vi "Check.vi"() -> ()   [LabVIEW 2023]
uses:
  <vilib>/DAQmx/read.llb/DAQmx Read (Digital Bool 1Line 1Point).vi
  <vilib>/DAQmx/write.llb/DAQmx Write (Digital Bool 1Line 1Point).vi
  <vilib>/DAQmx/read.llb/DAQmx Read (Digital 1D Bool NChan 1Samp 1Line).vi
  <vilib>/Utility/error.llb/Trim Whitespace One-Sided.vi
  <vilib>/DAQmx/create/channels.llb/DAQmx Create Channel (DO-Digital Output).vi
  <vilib>/DAQmx/create/channels.llb/DAQmx Create Channel (DI-Digital Input).vi
  <vilib>/Instr/_visa.llb/VISA Configure Serial Port (Instr).vi
  <vilib>/DAQmx/miscellaneous.llb/DAQmx Fill In Error Info.vi
panel:
  in  "VISA resource name":refnum<visa-resource-name>
  in  "Cry":tag
  in  "Motor":tag
  in  "Available":tag
  in  "Fan":tag
  in  "Wet":tag
  in  "Buzzer":tag
  in  "stop":bool
  in  "Cradle":bool
  out "read buffer":string
  out "Humidity":dbl(slide) scale=0.0..100.0
  out "Temperature":dbl(slide) scale=0.0..100.0
  out "Cry":bool
  out "Available":bool
  out "Wet":bool
  # "Input Output Panel"
  # "Indication Panel"
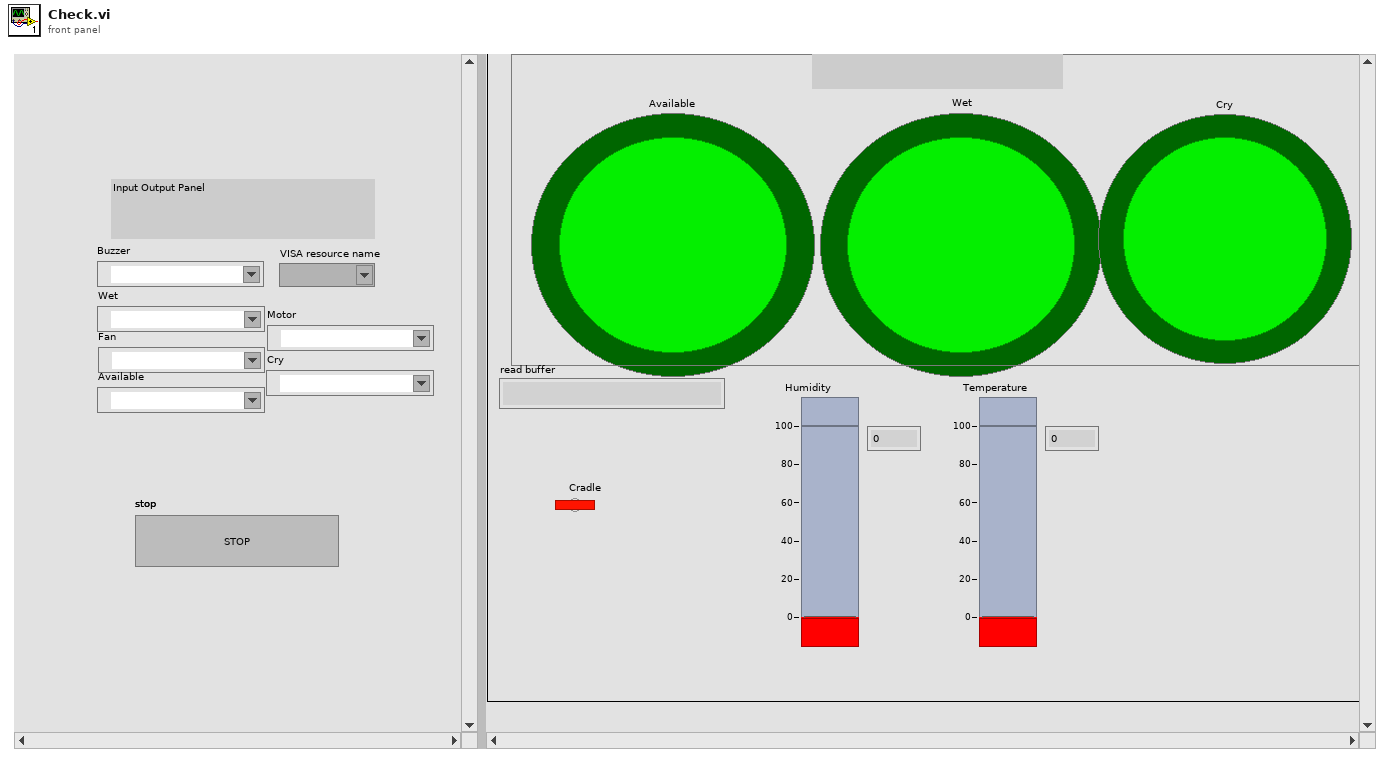
[diagram p1: front panel]
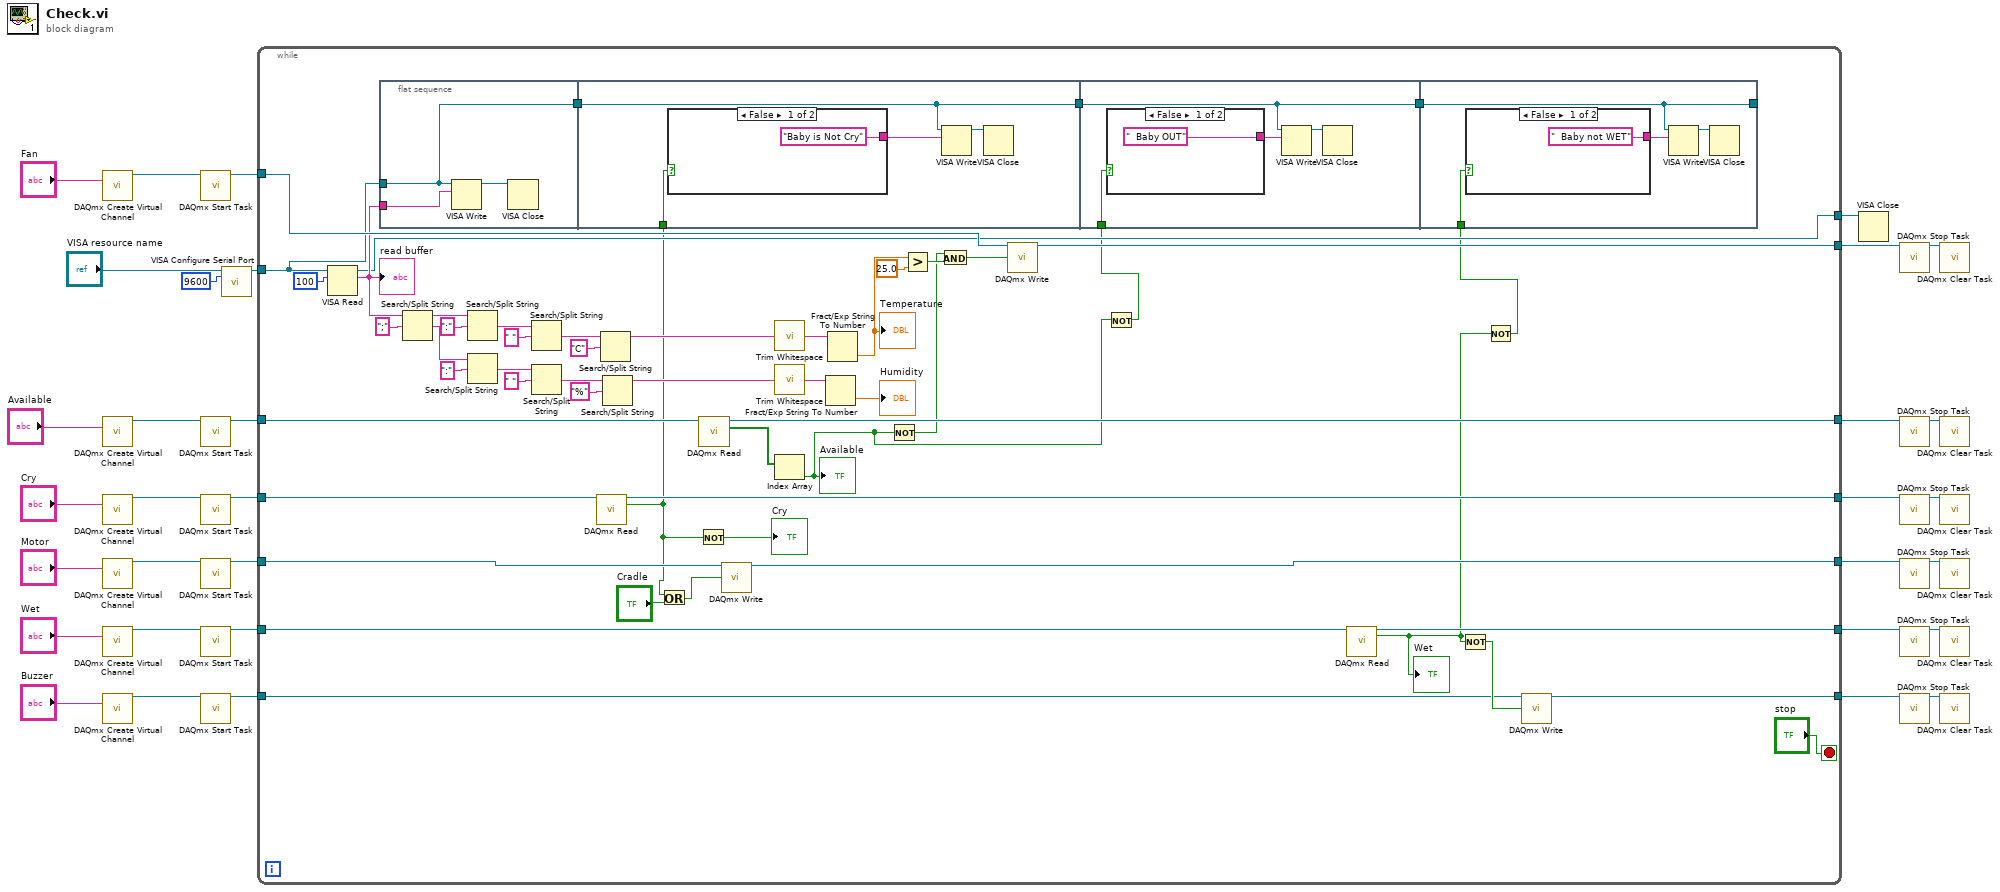
[diagram p0: block diagram]
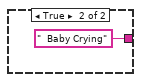
[diagram p2: hidden frame]
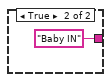
[diagram p3: hidden frame]
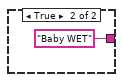
[diagram p4: hidden frame]
diagram:
  n1 = call-poly <vilib>:"DAQmx Create Virtual Channel.vi"("lines"="Fan") -> ("task out"=w21:refnum<k21>)  [unwired: 13 in, 1 out]
  n2 = call-poly <vilib>:"DAQmx Create Virtual Channel.vi"("lines"="Available") -> ("task out"=w18:refnum<k21>)  [unwired: 13 in, 1 out]
  n3 = call-poly <vilib>:"DAQmx Create Virtual Channel.vi"("lines"="Cry") -> ("task out"=w15:refnum<k21>)  [unwired: 13 in, 1 out]
  n4 = call-poly <vilib>:"DAQmx Create Virtual Channel.vi"("lines"="Motor") -> ("task out"=w12:refnum<k21>)  [unwired: 13 in, 1 out]
  n5 = call-poly <vilib>:"DAQmx Create Virtual Channel.vi"("lines"="Wet") -> ("task out"=w30:refnum<k21>)  [unwired: 13 in, 1 out]
  n6 = call-poly <vilib>:"DAQmx Create Virtual Channel.vi"("lines"="Buzzer") -> ("task out"=w34:refnum<k21>)  [unwired: 13 in, 1 out]
  n7 = call <vilib>:"DAQmx Start Task.vi"("task/channels in"=w21) -> ("task out"=w20:refnum<k21>)  [unwired: 13 in, 1 out]
  n8 = call <vilib>:"DAQmx Start Task.vi"("task/channels in"=w18) -> ("task out"=w17:refnum<k21>)  [unwired: 13 in, 1 out]
  n9 = call <vilib>:"DAQmx Start Task.vi"("task/channels in"=w15) -> ("task out"=w14:refnum<k21>)  [unwired: 13 in, 1 out]
  n10 = call <vilib>:"DAQmx Start Task.vi"("task/channels in"=w12) -> ("task out"=w11:refnum<k21>)  [unwired: 13 in, 1 out]
  n11 = call <vilib>:"DAQmx Start Task.vi"("task/channels in"=w30) -> ("task out"=w29:refnum<k21>)  [unwired: 13 in, 1 out]
  n12 = call <vilib>:"DAQmx Start Task.vi"("task/channels in"=w34) -> ("task out"=w2:refnum<k21>)  [unwired: 13 in, 1 out]
  n13 = call-poly "VISA Configure Serial Port"("VISA resource name"="VISA resource name", "baud rate (9600)"=u32 9600) -> ("VISA resource name out"=w4:refnum<visa-resource-name>)  [unwired: 12 in, 1 out]
  n14 = while {
    tunnel: w29 -> [w86]
    tunnel: [w85] -> w28
    tunnel: [w83] -> w24
    tunnel: [w82] -> w23
    tunnel: w20 -> [w81]
    tunnel: w17 -> [w80]
    tunnel: w14 -> [w79]
    tunnel: w11 -> [w78]
    tunnel: [w77] -> w9
    tunnel: [w76] -> w7
    tunnel: w4 -> [w50]
    tunnel: [w44] -> w3
    tunnel: w2 -> [w36]
    tunnel: [w35] -> w1
    stop <- "stop" stop-if-true
    n15 = VISA Read(VISA resource name=w50, byte count=u32 100) -> (VISA resource name out=w44:refnum<visa-resource-name>, read buffer=w60:string)  [unwired: 1 in, 2 out]
    "read buffer" <- w60
    n16 = flat-sequence {
      tunnel: w60 -> [w90]
      tunnel: [w88] -> w73
      tunnel: w50 -> [w88]
      tunnel: w73 -> [w93]
      tunnel: [w93] -> w72
      tunnel: w38 -> [w91]
      tunnel: w72 -> [w98]
      tunnel: [w98] -> w71
      tunnel: w42 -> [w97]
      tunnel: [w104] -> _
      tunnel: w71 -> [w104]
      tunnel: w40 -> [w103]
      frame #0 {
        n17 = VISA Write(VISA resource name=w88, write buffer=w90) -> (VISA resource name out=w89:refnum<visa-resource-name>)  [unwired: 1 in, 2 out]
        n18 = VISA Close(VISA resource name=w89) -> ()  [unwired: 1 in, 1 out]
      }
      frame #1 {
        n19 = case shown="False" w91 {
          tunnel: ["Baby is Not Cry" "  Baby Crying"] -> w94
          frame False {
          }
          frame True {
          }
        }
        n20 = VISA Write(VISA resource name=w93, write buffer=w94) -> (VISA resource name out=w92:refnum<visa-resource-name>)  [unwired: 1 in, 2 out]
        n21 = VISA Close(VISA resource name=w92) -> ()  [unwired: 1 in, 1 out]
      }
      frame #2 {
        n22 = case shown="False" w97 {
          tunnel: ["  Baby OUT" "Baby IN"] -> w100
          frame False {
          }
          frame True {
          }
        }
        n23 = VISA Write(VISA resource name=w98, write buffer=w100) -> (VISA resource name out=w99:refnum<visa-resource-name>)  [unwired: 1 in, 2 out]
        n24 = VISA Close(VISA resource name=w99) -> ()  [unwired: 1 in, 1 out]
      }
      frame #3 {
        n25 = case shown="False" w103 {
          tunnel: ["  Baby not WET" "Baby WET"] -> w106
          frame False {
          }
          frame True {
          }
        }
        n26 = VISA Write(VISA resource name=w104, write buffer=w106) -> (VISA resource name out=w105:refnum<visa-resource-name>)  [unwired: 1 in, 2 out]
        n27 = VISA Close(VISA resource name=w105) -> ()  [unwired: 1 in, 1 out]
      }
    }
    n28 = Search/Split String(string=w60, search string/char (-)=";") -> (substring before match=w68:string, match + rest of string=w51:string)  [unwired: 1 in, 1 out]
    n29 = Search/Split String(string=w68, search string/char (-)=":") -> (match + rest of string=w65:string)  [unwired: 1 in, 2 out]
    n30 = Search/Split String(string=w51, search string/char (-)=":") -> (match + rest of string=w57:string)  [unwired: 1 in, 2 out]
    n31 = Search/Split String(string=w65, search string/char (-)=" ") -> (match + rest of string=w63:string)  [unwired: 1 in, 2 out]
    n32 = Search/Split String(string=w57, search string/char (-)=" ") -> (match + rest of string=w55:string)  [unwired: 1 in, 2 out]
    n33 = call-poly <vilib>:"DAQmx Read.vi"("task/channels in"=w79) -> ("task out"=w77:refnum<k21>, "data"=w38:bool)  [unwired: 12 in, 1 out]
    n34 = Search/Split String(string=w63, search string/char (-)="C") -> (substring before match=w62:string)  [unwired: 1 in, 2 out]
    n35 = Search/Split String(string=w55, search string/char (-)="%") -> (substring before match=w54:string)  [unwired: 1 in, 2 out]
    n36 = Or(x=w38, y="Cradle") -> (x .or. y?=w39:bool)
    n37 = Not(x=w38) -> (.not. x?=→"Cry":bool)
    n38 = call-poly <vilib>:"DAQmx Read.vi"("task/channels in"=w80) -> ("task out"=w82:refnum<k21>, "data"=w75:bool[])  [unwired: 12 in, 1 out]
    n39 = call-poly <vilib>:"DAQmx Write.vi"("task/channels in"=w78, "data"=w39) -> ("task out"=w76:refnum<k21>)  [unwired: 11 in, 2 out]
    n40 = call <vilib>:"Trim Whitespace.vi"("string"=w62) -> ("trimmed string"=w61:string)  [unwired: 1 in]
    n41 = call <vilib>:"Trim Whitespace.vi"("string"=w54) -> ("trimmed string"=w53:string)  [unwired: 1 in]
    n42 = Index Array(array=w75) -> (element=w43:bool)  [unwired: 1 in]
    "Available" <- w43
    n43 = Fract/Exp String To Number(string=w53) -> (number=→"Humidity":dbl)  [unwired: 3 in, 1 out]
    n44 = Fract/Exp String To Number(string=w61) -> (number=w48:dbl)  [unwired: 3 in, 1 out]
    "Temperature" <- w48
    n45 = Not(x=w43) -> (.not. x?=w46:bool)
    n46 = Greater?(x=w48, y=25.0) -> (0:w47:bool)
    n47 = And(x=w46, y=w47) -> (x .and. y?=w45:bool)
    n48 = call-poly <vilib>:"DAQmx Write.vi"("task/channels in"=w81, "data"=w45) -> ("task out"=w83:refnum<k21>)  [unwired: 11 in, 2 out]
    n49 = Not(x=w43) -> (.not. x?=w42:bool)
    n50 = call-poly <vilib>:"DAQmx Read.vi"("task/channels in"=w86) -> ("task out"=w85:refnum<k21>, "data"=w41:bool)  [unwired: 12 in, 1 out]
    "Wet" <- w41
    n51 = Not(x=w41) -> (.not. x?=w84:bool)
    n52 = Not(x=w41) -> (.not. x?=w40:bool)
    n53 = call-poly <vilib>:"DAQmx Write.vi"("task/channels in"=w36, "data"=w84) -> ("task out"=w35:refnum<k21>)  [unwired: 11 in, 2 out]
  }
  n54 = VISA Close(VISA resource name=w3) -> ()  [unwired: 1 in, 1 out]
  n55 = call <vilib>:"DAQmx Stop Task.vi"("task/channels in"=w24) -> ("task out"=w25:refnum<k21>)  [unwired: 13 in, 1 out]
  n56 = call <vilib>:"DAQmx Stop Task.vi"("task/channels in"=w23) -> ("task out"=w26:refnum<k21>)  [unwired: 13 in, 1 out]
  n57 = call <vilib>:"DAQmx Stop Task.vi"("task/channels in"=w9) -> ("task out"=w8:refnum<k21>)  [unwired: 13 in, 1 out]
  n58 = call <vilib>:"DAQmx Stop Task.vi"("task/channels in"=w7) -> ("task out"=w10:refnum<k21>)  [unwired: 13 in, 1 out]
  n59 = call <vilib>:"DAQmx Stop Task.vi"("task/channels in"=w28) -> ("task out"=w27:refnum<k21>)  [unwired: 13 in, 1 out]
  n60 = call <vilib>:"DAQmx Stop Task.vi"("task/channels in"=w1) -> ("task out"=w33:refnum<k21>)  [unwired: 13 in, 1 out]
  n61 = call <vilib>:"DAQmx Clear Task.vi"("task in"=w25) -> ()  [unwired: 14 in, 1 out]
  n62 = call <vilib>:"DAQmx Clear Task.vi"("task in"=w26) -> ()  [unwired: 14 in, 1 out]
  n63 = call <vilib>:"DAQmx Clear Task.vi"("task in"=w8) -> ()  [unwired: 14 in, 1 out]
  n64 = call <vilib>:"DAQmx Clear Task.vi"("task in"=w10) -> ()  [unwired: 14 in, 1 out]
  n65 = call <vilib>:"DAQmx Clear Task.vi"("task in"=w27) -> ()  [unwired: 14 in, 1 out]
  n66 = call <vilib>:"DAQmx Clear Task.vi"("task in"=w33) -> ()  [unwired: 14 in, 1 out]
